vi "RANGE Check Standard Gas.vi"(11 "Gas Type":string) -> (2 "Standard Gas":bool, 3 "Gas Type":string)   [LabVIEW 2018]
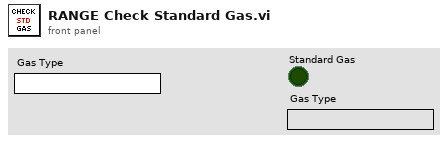
[diagram p1: front panel]
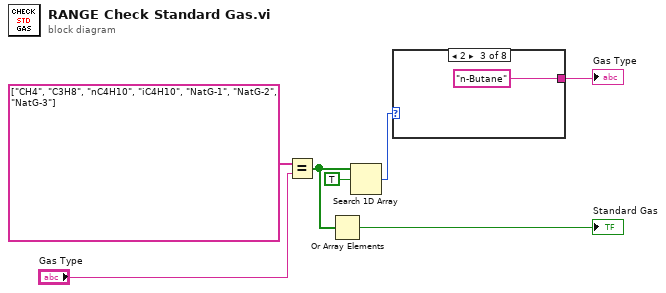
[diagram p0: block diagram]
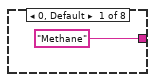
[diagram p2: hidden frame]
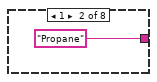
[diagram p3: hidden frame]
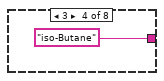
[diagram p4: hidden frame]
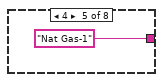
[diagram p5: hidden frame]
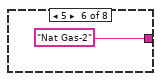
[diagram p6: hidden frame]
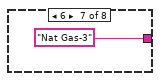
[diagram p7: hidden frame]
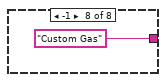
[diagram p8: hidden frame]
diagram:
  n1 = Equal?(x=string[] ["CH4", "C3H8", "nC4H10", "iC4H10", "NatG-1", "NatG-2", "NatG-3"], y="Gas Type") -> (x = y?=w4:bool[])
  n2 = Or Array Elements(Boolean array=w4) -> (logical OR=→"Standard Gas":bool)
  n3 = Search 1D Array(1D array=w4, element=TRUE) -> (index of element=w2:i32)  [unwired: 1 in]
  n4 = case shown="2" w2 {
    tunnel: ["Methane" "Propane" "n-Butane" "iso-Butane" "Nat Gas-1" "Nat Gas-2" "Nat Gas-3" "Custom Gas"] -> w1
    frame 0, Default {
    }
    frame 1 {
    }
    frame 2 {
    }
    frame 3 {
    }
    frame 4 {
    }
    frame 5 {
    }
    frame 6 {
    }
    frame -1 {
    }
  }
  "Gas Type" <- w1
